vi "picoquant_process_records.vi"(8 "error in (no error)":errorcluster, 10 "data":u32[](array[numeric]), 11 "picoquant_generic in":refnum<class "picoquant_generic.lvclass">) -> (0 "error out":errorcluster, 2 "data 2":T1, 3 "picoquant_generic out":refnum<class "picoquant_generic.lvclass">)   [LabVIEW 2015, in "picoquant_generic.lvclass"]
uses:
  picoquant_generic.lvclass
  picoquant_data_tdef.ctl
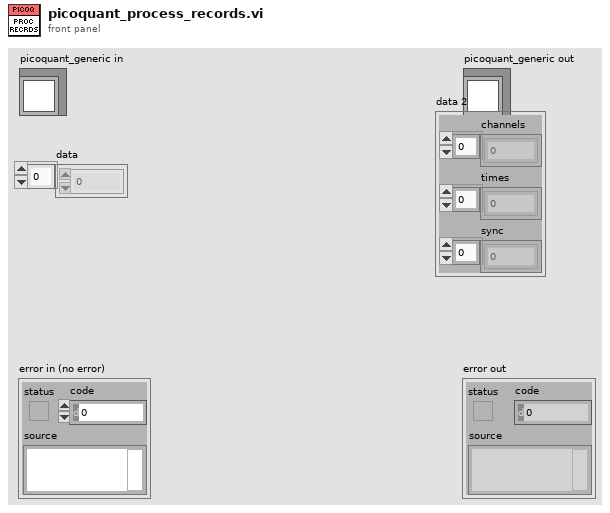
[diagram p1: front panel]
types:
  T1 = typedef "picoquant_data_tdef.ctl" = cluster{"channels":u8[], "times":u64[], "sync":u64[]}
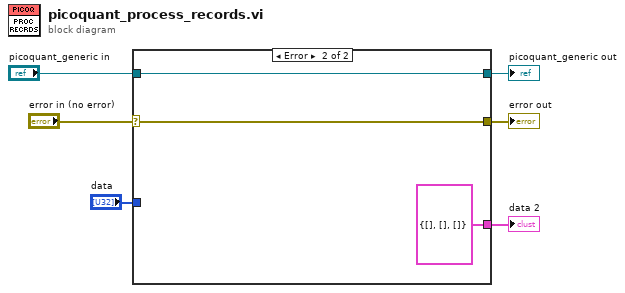
[diagram p0: block diagram]
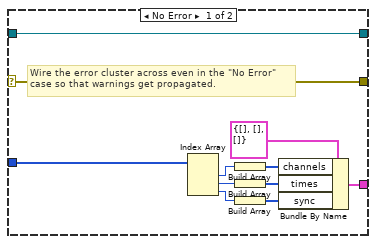
[diagram p2: hidden frame]
diagram:
  n1 = case shown="Error" "error in (no error)" {
    selector: "error in (no error)" -> [w16 w20]
    tunnel: [w16 w20] -> w5
    tunnel: [w17 w19] -> w3
    tunnel: "picoquant_generic in" -> [w17 w19]
    tunnel: "data" -> [w13 _]
    tunnel: [w14 T1 {"channels"=[], "times"=[], "sync"=[]} ("data 2")] -> w1
    frame No Error {
      # "Wire the error cluster across even in the \"No Error\"\ncase so that warnings get propagated."
      n2 = Index Array(array=w13) -> (element #1=w10:u32, element #2=w11:u32, element #3=w12:u32)  [unwired: 3 in]
      n3 = Build Array(w10) -> (w9:u32[])
      n4 = Build Array(w11) -> (w8:u32[])
      n5 = Build Array(w12) -> (w7:u32[])
      n6 = Bundle By Name(cluster=T1 {"channels"=[], "times"=[], "sync"=[]} ("data 2"), "channels"=w9, "times"=w8, "sync"=w7) -> (w14:T1)
    }
    frame Error {
    }
  }
  "error out" <- w5
  "picoquant_generic out" <- w3
  "data 2" <- w1
